vi "Init Actor Core.vi"(8 "error in (no error)":errorcluster, 11 "Monitor-Pulse in":refnum<class "Monitor-Pulse.lvclass">) -> (0 "error out":errorcluster, 3 "Monitor-Pulse out":refnum<class "Monitor-Pulse.lvclass">)   [LabVIEW 2015, in "Monitor-Pulse.lvclass"]
uses:
  Monitor-Pulse.lvclass
  Measure_core/Measure Controller/Measure Controller.lvclass/Measure Controller.ctl
  Monitor-Pulse.lvclass/Monitor-Pulse.ctl
  Measure_core/Pulse Controller/Pulse Controller.lvclass
  Measure_core/Controllers/Monitor Controller/Monitor Controller.lvclass
  Post-Processors/Integrate/Integrate.lvclass
  <vilib>/ActorFramework/Actor/Actor.lvclass/Actor.ctl
  <vilib>/ActorFramework/Message Enqueuer/Message Enqueuer.lvclass/Message Enqueuer.ctl
  <vilib>/ActorFramework/Message Enqueuer/Init from Existing Queue.vi
  <vilib>/ActorFramework/Message Enqueuer/Enqueue.vi
  <vilib>/ActorFramework/Message Priority Queue/Priority Enqueue.vi
  <vilib>/ActorFramework/Message Enqueuer/Message Enqueuer.lvclass
  Measure_core/Measure Object Messages/Open Front Panel Msg/Open Front Panel Msg.lvclass
  Measure_core/Measure Controller/Measure Controller.lvclass
  <vilib>/ActorFramework/Actor/Actor.lvclass
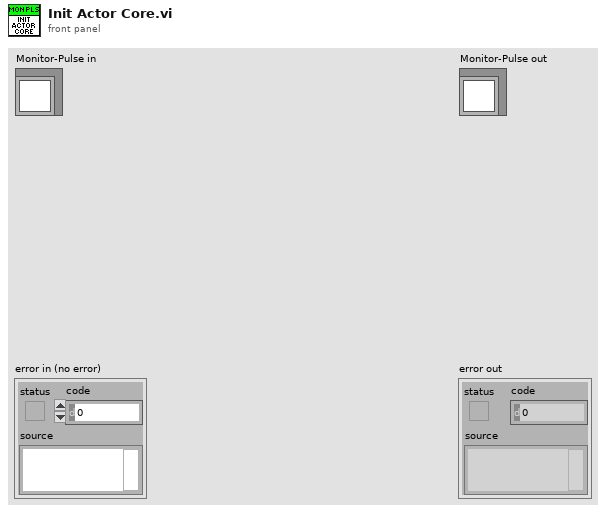
[diagram p1: front panel]
types:
  T1 = typedef "Module Types.ctl" = enum16{"NONE", "NI-DAQmx", "NI-Scope", "Red Pitaya Digitizer", "GaGe", "VISA Device", "Red Piataya Lockin", "Monitor Controller", "Pulse Controller", "Integrate Pulse"}
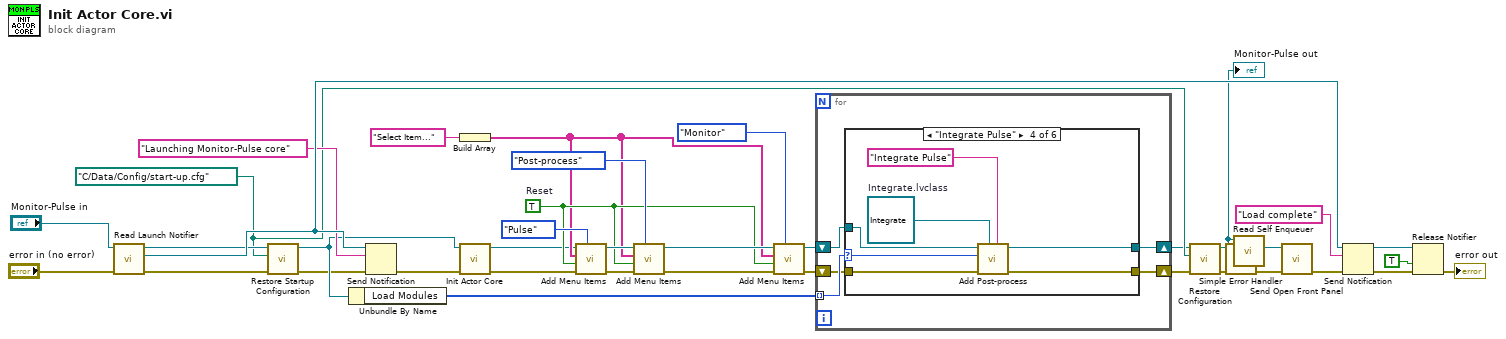
[diagram p0: block diagram]
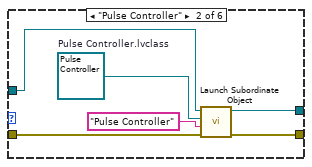
[diagram p3: hidden frame]
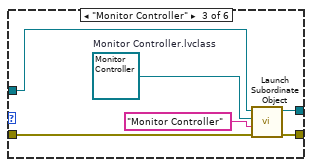
[diagram p4: hidden frame]
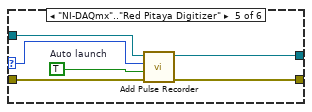
[diagram p5: hidden frame]
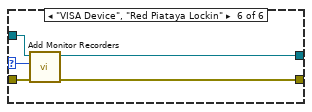
[diagram p6: hidden frame]
diagram:
  w6 = path "C:/Data/Config/start-up.cfg" ("Startup Configuration File")
  w24 = TRUE  # Reset
  n1 = call "Read Launch Notifier.vi"("error in (no error)"="error in (no error)", "Measure Controller in"="Monitor-Pulse in") -> ("error out"=w9:errorcluster, "Launch Notifier"=w18:refnum<notifier>, "Measure Controller out"=w10:refnum<class "Monitor-Pulse.lvclass">)  [unwired: 7 in]
  n2 = call-dynamic "Restore Startup Configuration.vi"("error in (no error)"=w9, "Startup Configuration File"=w6, "Monitor-Pulse in"=w10) -> ("error out"=w7:errorcluster, "Monitor-Pulse out"=w8:refnum<class "Monitor-Pulse.lvclass">)  [unwired: 7 in]
  n3 = Unbundle By Name(w8) -> ("Load Modules"=w16:T1[])
  n4 = Send Notification(notification="Launching Monitor-Pulse core", notifier=w18, error in (no error)=w7) -> (error out=w19:errorcluster)  [unwired: 1 out]
  n5 = Build Array("Select Item..." ("element")) -> (w15:string[])
  n6 = call-parent "Init Actor Core.vi"("error in (no error)"=w19, "Measure Object in"=w8) -> ("error out"=w11:errorcluster, "Measure Object out"=w13:refnum<class "Monitor-Pulse.lvclass">)  [unwired: 8 in]
  n7 = call-dynamic "Add Menu Items.vi"("Menu control"=enum16{"Pulse", "Post-process", "Monitor"}."Pulse", "error in (no error)"=w11, "Reset"=w24, "Item Names"=w15, "Monitor-Pulse in"=w13) -> ("error out"=w30:errorcluster, "Monitor-Pulse out"=w32:refnum<class "Monitor-Pulse.lvclass">)  [unwired: 5 in]
  n8 = call-dynamic "Add Menu Items.vi"("Menu control"=enum16{"Pulse", "Post-process", "Monitor"}."Post-process", "error in (no error)"=w30, "Reset"=w24, "Item Names"=w15, "Monitor-Pulse in"=w32) -> ("error out"=w26:errorcluster, "Monitor-Pulse out"=w27:refnum<class "Monitor-Pulse.lvclass">)  [unwired: 5 in]
  n9 = call-dynamic "Add Menu Items.vi"("Menu control"=enum16{"Pulse", "Post-process", "Monitor"}."Monitor", "error in (no error)"=w26, "Reset"=w24, "Item Names"=w15, "Monitor-Pulse in"=w27) -> ("error out"=w14:errorcluster, "Monitor-Pulse out"=w12:refnum<class "Monitor-Pulse.lvclass">)  [unwired: 5 in]
  n10 = for {
    tunnel: w16 -> [w42] mode=indexing
    shift-right: [w40] -> w3
    shift-left: w14 -> [w41]
    shift-right: [w38] -> w5
    shift-left: w12 -> [w39]
    n11 = case shown="\"Integrate Pulse\"" w42 {
      selector: w42 -> [_ _ _ w57 w69 w70]
      tunnel: w41 -> [w43 w46 w54 w59 w67 w74]
      tunnel: [w43 w45 w53 w58 w66 w73] -> w40
      tunnel: w39 -> [w44 w48 w56 w63 w65 w72]
      tunnel: [w44 w47 w55 w62 w64 w71] -> w38
      frame "NONE", Default {
      }
      frame "Pulse Controller" {
        w49 = refnum<class "Pulse Controller.lvclass"> refnum  # Pulse Controller.lvclass
        n12 = call-dynamic "Launch Subordinate Object.vi"("error in (no error)"=w46, "Name"="Pulse Controller", "Subordinate Object"=w49, "Measure Object in"=w48) -> ("error out"=w45:errorcluster, "Measure Object out"=w47:refnum<class "Monitor-Pulse.lvclass">)  [unwired: 5 in, 1 out]
      }
      frame "Monitor Controller" {
        w52 = refnum<class "Monitor Controller.lvclass"> refnum  # Monitor Controller.lvclass
        n13 = call-dynamic "Launch Subordinate Object.vi"("error in (no error)"=w54, "Name"="Monitor Controller", "Subordinate Object"=w52, "Measure Object in"=w56) -> ("error out"=w53:errorcluster, "Measure Object out"=w55:refnum<class "Monitor-Pulse.lvclass">)  [unwired: 5 in, 1 out]
      }
      frame "Integrate Pulse" {
        w61 = refnum<class "Integrate.lvclass"> refnum  # Integrate.lvclass
        n14 = call-dynamic "Add Post-process.vi"("Name"="Integrate Pulse", "Subordinate Object"=w61, "error in (no error)"=w59, "Module type"=w57, "Monitor-Pulse in"=w63) -> ("error out"=w58:errorcluster, "Monitor-Pulse out"=w62:refnum<class "Monitor-Pulse.lvclass">)  [unwired: 5 in]
      }
      frame "NI-DAQmx".."Red Pitaya Digitizer" {
        w68 = TRUE  # Auto launch
        n15 = call-dynamic "Add Pulse Recorder.vi"("error in (no error)"=w67, "Auto launch"=w68, "Module type"=w69, "Monitor-Pulse in"=w65) -> ("error out"=w66:errorcluster, "Monitor-Pulse out"=w64:refnum<class "Monitor-Pulse.lvclass">)  [unwired: 6 in]
      }
      frame "VISA Device", "Red Piataya Lockin" {
        n16 = call-dynamic "Add Monitor Recorders.vi"("error in (no error)"=w74, "Module type"=w70, "Monitor-Pulse in"=w72) -> ("error out"=w73:errorcluster, "Monitor-Pulse out"=w71:refnum<class "Monitor-Pulse.lvclass">)  [unwired: 6 in, 1 out]
      }
    }
  }
  n17 = call-dynamic "Restore Configuration.vi"("error in (no error)"=w3, "File path"=w6, "Monitor-Pulse in"=w5) -> ("error out"=w2:errorcluster, "Monitor-Pulse out"=w4:refnum<class "Monitor-Pulse.lvclass">)  [unwired: 5 in, 2 out]
  "Monitor-Pulse out" <- w4
  n18 = call <vilib>:"Simple Error Handler.vi"("error in (no error)"=w2) -> ("error out"=w1:errorcluster)  [unwired: 4 in, 4 out]
  n19 = call <vilib>:"Read Self Enqueuer.vi"("Actor"=w4) -> ("Self Enqueuer"=w37:refnum<class "Message Enqueuer.lvclass">)  [unwired: 10 in]
  n20 = call "Send Open Front Panel.vi"("error in (no error)"=w1, "Message Enqueuer"=w37) -> ("error out"=w22:errorcluster)  [unwired: 8 in, 1 out]
  n21 = Send Notification(notification="Load complete" ("Message"), notifier=w18, error in (no error)=w22) -> (notifier out=w34:refnum<notifier>, error out=w35:errorcluster)
  n22 = Release Notifier(notifier=w34, force destroy? (F)=TRUE ("Kill notifier"), error in (no error)=w35) -> (error out=→"error out":errorcluster)  [unwired: 2 out]
